vi "e1039-target-heattape-read-SubVI.vi"() -> ()   [LabVIEW 2019]
uses:
  <vilib>/NI/Modbus Library/API/Wrapper/Create Serial Master.vi
  <vilib>/NI/Modbus Library/API/Master/Modbus Master.lvclass
  <vilib>/NI/Modbus Library/API/Wrapper/API Main.lvlib
panel:
  in  "Set Value (Station 01)":string
  out "Numeric":dbl
  out "String 2":string
  in  "error check 2":errorcluster
  in  "COM Port (Station 02)":refnum<visa-resource-name>
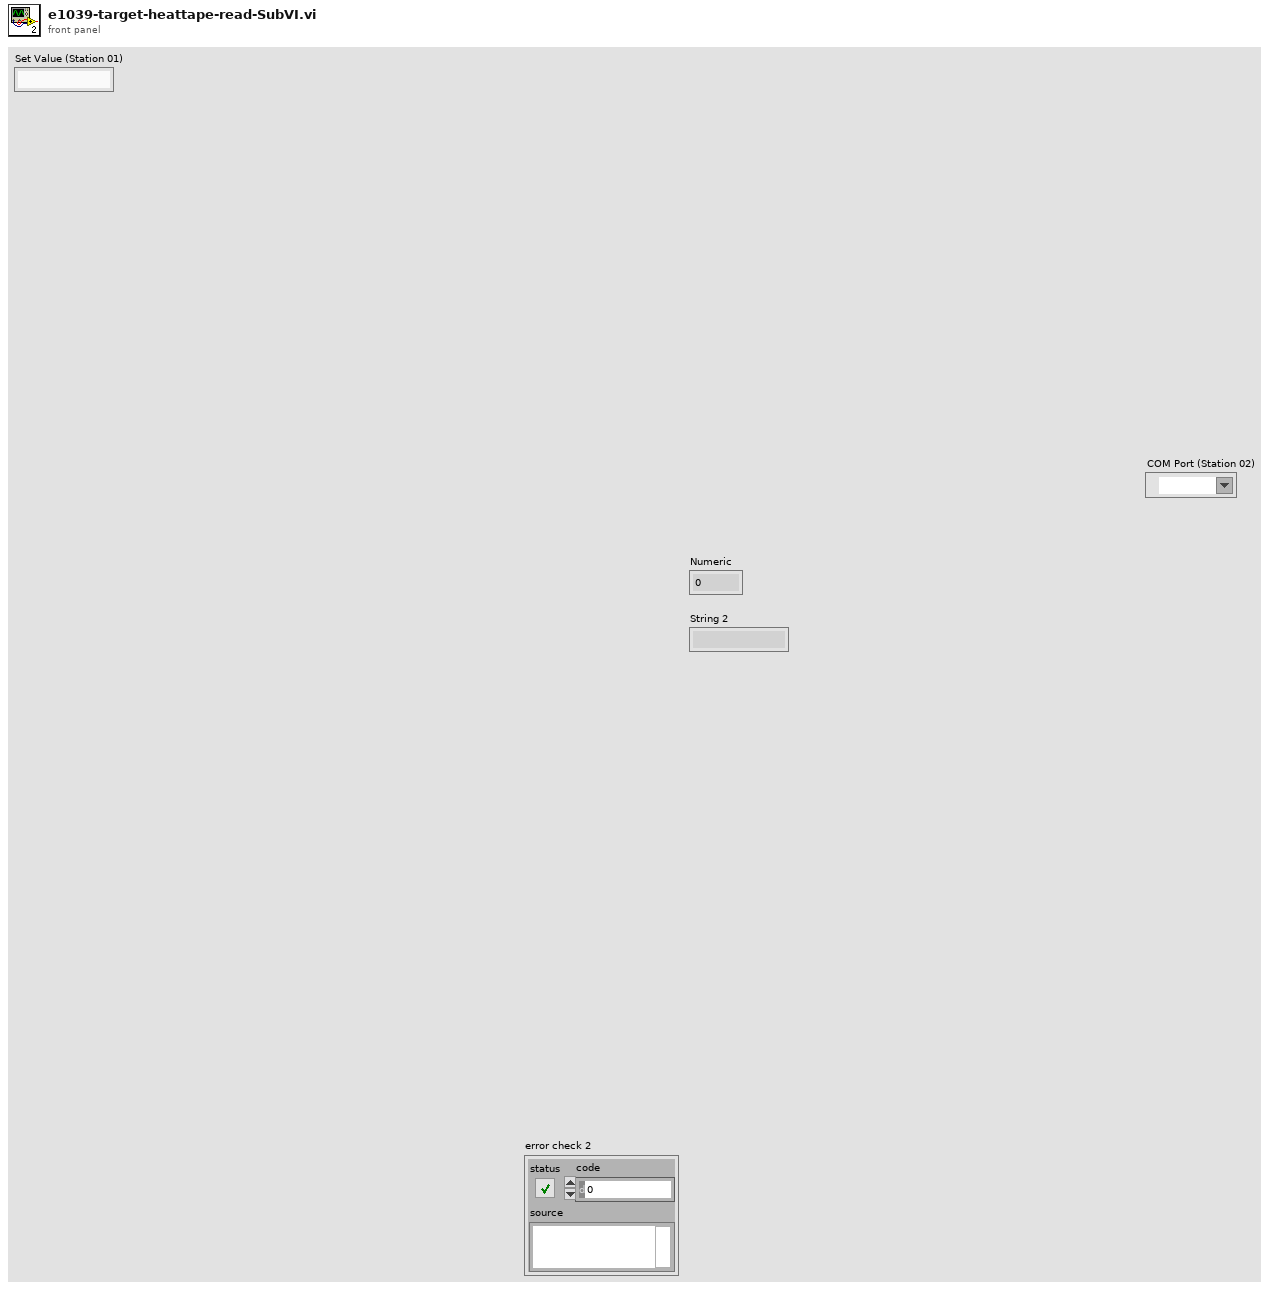
[diagram p1: front panel]
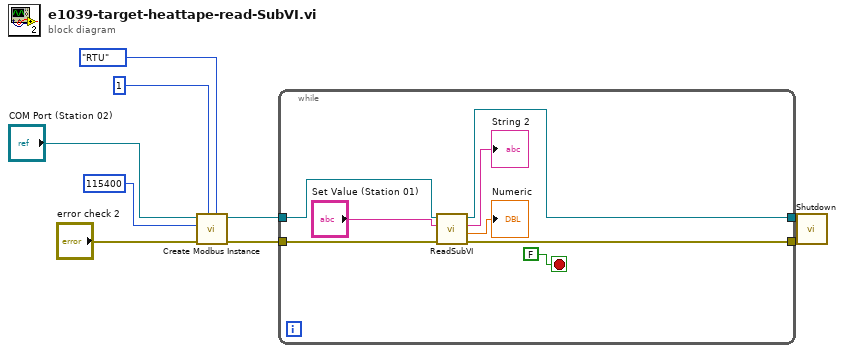
[diagram p0: block diagram]
diagram:
  n1 = call-poly <vilib>:"Create Modbus Instance.vi"("serial type"=enum16{"RTU", "ASCII"}."RTU" ("Serial Type (Default: RTU)"), "unit ID"=u8 1 ("unit ID (Defaut: 1)"), "error in"="error check 2", "baud rate"=u32 115400 ("Baud Rate (Default: 115400)"), "VISA resource name"="COM Port (Station 02)") -> ("error out"=w3:errorcluster, "serial master instance"=w4:refnum<class "Modbus Master.lvclass">)  [unwired: 5 in]
  n2 = while {
    tunnel: w4 -> [w17]
    tunnel: w3 -> [w16]
    tunnel: [w15] -> w2
    tunnel: [w14] -> w1
    stop <- FALSE stop-if-true
    n3 = call "ReadSubVI.vi"("error in (no error)"=w16, "Set Value (Station 01)"="Set Value (Station 01)", "Modbus Master in"=w17) -> ("error out"=w15:errorcluster, "Numeric"=→"Numeric":dbl, "String"=→"String 2":string, "Modbus Master out"=w14:refnum<class "Modbus Master.lvclass">)  [unwired: 5 in]
  }
  n4 = call-dynamic "Shutdown.vi"("error in"=w2, "Modbus master in"=w1) -> ()  [unwired: 9 in, 1 out]
